vi "Subdevide.vi"(0 "Input String":string, 1 "Delimiter":string=" ") -> (2 "Output Array":string[](array[string]))   [LabVIEW 2011]
doc: "This VI subdevide a string to an array with space as a delimiter."
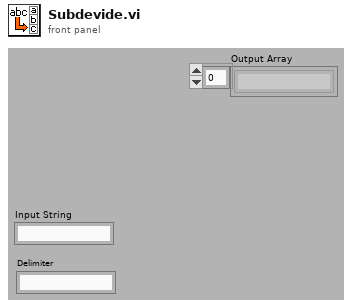
[diagram p1: front panel]
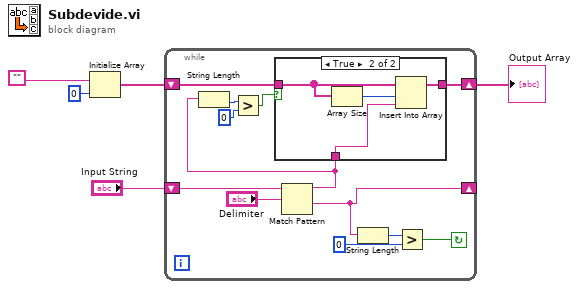
[diagram p0: block diagram]
diagram:
  n1 = Initialize Array("", 0 ("dimension size")) -> (w4:string[])
  n2 = while {
    shift-right: [w17] -> w1
    shift-left: w4 -> [w16]
    shift-right: [w13] -> _
    shift-left: "Input String" -> [w15]
    stop <- w11 continue-if-true
    n3 = Match Pattern(string=w15, regular expression="Delimiter") -> (before substring=w6:string, after substring=w13:string)  [unwired: 1 in, 2 out]
    n4 = String Length(string=w6) -> (length=w9:i32)
    n5 = Greater?(x=w9, y=0) -> (0:w8:bool)
    n6 = case shown="True" w8 {
      tunnel: [w18 w22] -> w17
      tunnel: w16 -> [w18 w21]
      tunnel: w6 -> [_ w19]
      frame False {
      }
      frame True {
        n7 = Array Size(array=w21) -> (size(s)=w20:i32)
        n8 = Insert Into Array(array=w21, index=w20, new element=w19) -> (w22:string[])
      }
    }
    n9 = String Length(string=w13) -> (length=w14:i32)
    n10 = Greater?(x=w14, y=0) -> (0:w11:bool)
  }
  "Output Array" <- w1
